vi "Read Data Path.vi"(8 "error in (no error)":errorcluster, 11 "Configuration File In":refnum<class "Configuration File.lvclass">) -> (0 "error out":errorcluster, 1 "value":path, 3 "Configuration File Out":refnum<class "Configuration File.lvclass">)   [LabVIEW 2020, in "Configuration File.lvclass"]
doc: "High-level function for reading configuration file data from process class."
uses:
  Configuration File.lvclass
  <vilib>/Utility/config.llb/Read Key (Path).vi
  <vilib>/Utility/config.llb/Write Key (Path).vi
  <vilib>/Utility/config.llb/NI_LVConfig.lvlib
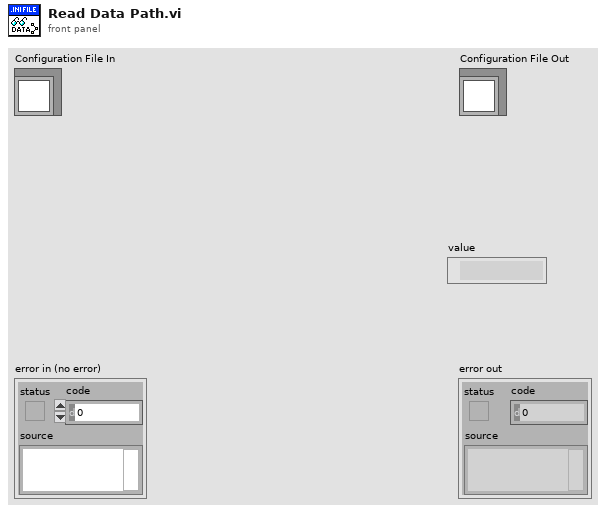
[diagram p1: front panel]
types:
  T1 = typedef "NI_LVConfig.lvlib/Config Data RefNum.ctl" = refnum<k1>
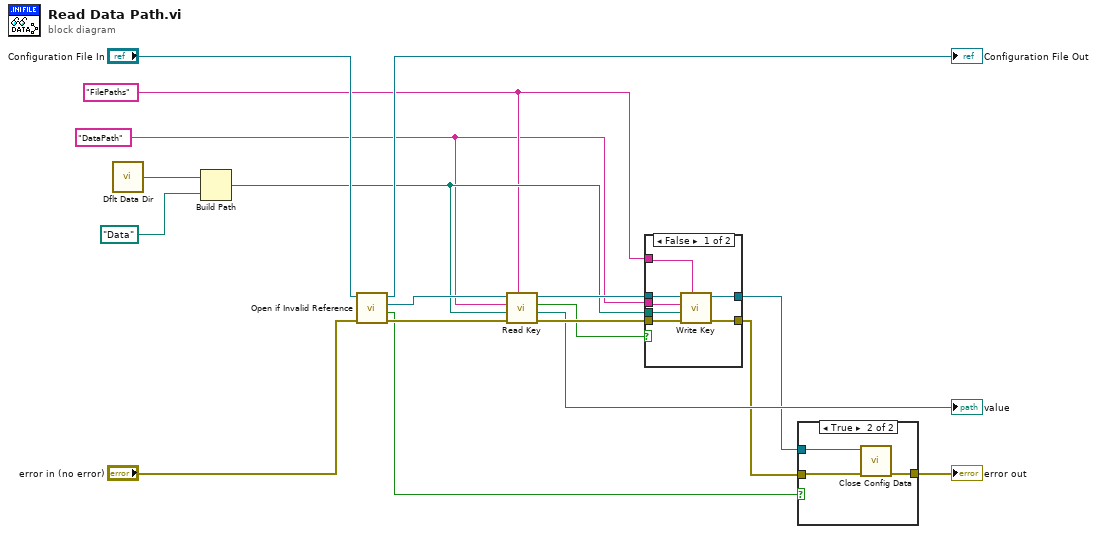
[diagram p0: block diagram]
diagram:
  w1 = "DataPath" ("Process Name")
  w2 = "FilePaths" ("Process Name")
  n1 = call <vilib>:"Dflt Data Dir.vi"() -> ("App:Default Data Directory"=w3:path)
  n2 = Build Path(base path=w3, name or relative path=path "Data" ("default value")) -> (appended path=w4:path)
  n3 = call "Open if Invalid Reference.vi"("error in (no error)"="error in (no error)", "Configuration File In"="Configuration File In") -> ("error out"=w10:errorcluster, "File opened?"=w5:bool, "refnum out"=w11:T1, "Configuration File Out"=→"Configuration File Out":refnum<class "Configuration File.lvclass">)  [unwired: 6 in]
  n4 = call-poly <vilib>:"Read Key.vi"("section"=w2, "error in (no error)"=w10, "default value"=w4, "key"=w1, "refnum"=w11) -> ("error out"=w16:errorcluster, "value"=→"value":path, "found?"=w15:bool, "refnum out"=w17:T1)  [unwired: 3 in]
  n5 = case shown="False" w15 {
    tunnel: w17 -> [w25 w27]
    tunnel: w16 -> [w24 w26]
    tunnel: [w23 w27] -> w8
    tunnel: [w22 w26] -> w7
    tunnel: w1 -> [w21 _]
    tunnel: w2 -> [w20 _]
    tunnel: w4 -> [w19 _]
    frame False {
      n6 = call-poly <vilib>:"Write Key.vi"("section"=w20, "error in (no error)"=w24, "value"=w19, "key"=w21, "refnum"=w25) -> ("error out"=w22:errorcluster, "refnum out"=w23:T1)  [unwired: 4 in, 1 out]
    }
    frame True {
    }
  }
  n7 = case shown="True" w5 {
    tunnel: w8 -> [_ w31]
    tunnel: w7 -> [w28 w30]
    tunnel: [w28 w29] -> w6
    frame False {
    }
    frame True {
      n8 = call <vilib>:"Close Config Data.vi"("error in (no error)"=w30, "refnum"=w31) -> ("error out"=w29:errorcluster)  [unwired: 8 in, 1 out]
    }
  }
  "error out" <- w6
